vi "LEP_RV_SaveDebugMode.vi"(8 "error in":errorcluster) -> (0 "error out":errorcluster)   [LabVIEW 2011]
uses:
  <vilib>/Platform/EmbProject/Plugins/utilities/LEP_Utilities_GetSetProjectData_Variant.vi
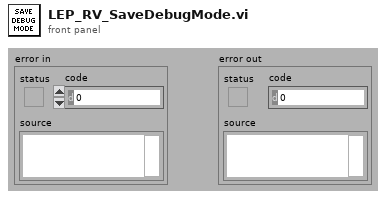
[diagram p1: front panel]
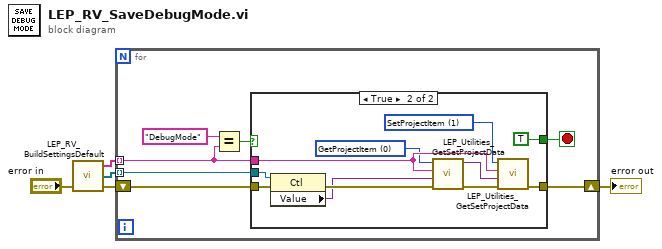
[diagram p0: block diagram]
diagram:
  n1 = call "LEP_RV_BuildSettingsDefault.vi"("error in (no error)"="error in") -> ("error out"=w3:errorcluster, "Default Values"=w2:refnum<vi>[], "Attribute Name"=w1:string[])  [unwired: 2 out]
  n2 = for {
    shift-right: [w7] -> w5
    shift-left: w3 -> [w8]
    tunnel: w2 -> [w10] mode=indexing
    tunnel: w1 -> [w11] mode=indexing
    stop <- w6 stop-if-true
    n3 = Equal?(x="DebugMode", y=w11) -> (x = y?=w9:bool)
    n4 = case shown="True" w9 {
      tunnel: w11 -> [_ w18]
      tunnel: w10 -> [_ w19]
      tunnel: w8 -> [w13 w16]
      tunnel: [w13 w15] -> w7
      tunnel: [_ TRUE] -> w6
      frame False {
      }
      frame True {
        w17 = u16 0 items=["GetProjectItem", "SetProjectItem"] ("Command")
        w22 = u16 1 items=["GetProjectItem", "SetProjectItem"] ("Command")
        n5 = property class="Ctl"(reference=w19, error in=w16) -> (error out=w24:errorcluster, "Value"=w23:variant)  [unwired: 1 out]
        n6 = call-poly <vilib>:"LEP_Utilities_GetSetProjectData.vi"("error in"=w24, "Variant In"=w23, "ItemName"=w18, "Command"=w17) -> ("error out"=w21:errorcluster, "Variant Out"=w20:variant)  [unwired: 1 in, 5 out]
        n7 = call-poly <vilib>:"LEP_Utilities_GetSetProjectData.vi"("error in"=w21, "Variant In"=w20, "ItemName"=w18, "Command"=w22) -> ("error out"=w15:errorcluster)  [unwired: 1 in, 6 out]
      }
    }
  }
  "error out" <- w5
